vi "Decimate calc factors.vi"(9 "display width":i32, 11 "input buffer size":i32) -> (1 "decimation factor":i32, 2 "no decimation?":bool, 3 "output buffer size":i32)   [LabVIEW 2021, in "RocketPlot.lvlib"]
uses:
  RocketPlot.lvlib
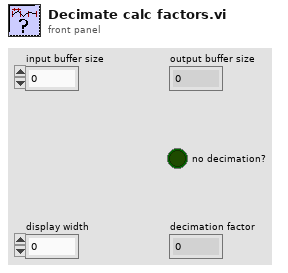
[diagram p1: front panel]
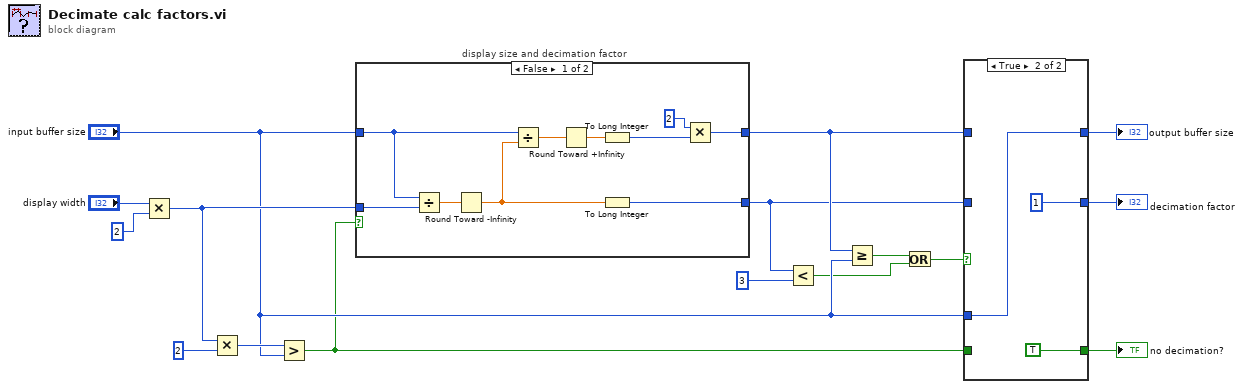
[diagram p0: block diagram]
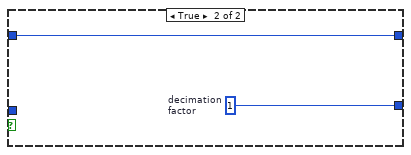
[diagram p2: hidden frame]
diagram:
  n1 = Multiply(x="display width", y=2) -> (x*y=w16:i32)
  n2 = Multiply(x=w16, y=2 ("x")) -> (x*y=w15:i32)
  n3 = Greater?(x=w15, y="input buffer size") -> (0:w1:bool)
  n4 = case "display size and decimation factor" shown="False" w1 {
    tunnel: "input buffer size" -> [w17 w28]
    tunnel: w16 -> [w26 _]
    tunnel: [w19 w28] -> w10
    tunnel: [w24 w27] -> w6
    frame False {
      n5 = Divide(x=w17, y=w26) -> (x/y=w25:dbl)
      n6 = Round Toward -Infinity(1:w25) -> (0:w23:dbl)
      n7 = Divide(x=w17, y=w23) -> (x/y=w22:dbl)
      n8 = Round Toward +Infinity(x=w22) -> (ceil(x): smallest int >= x=w21:dbl)
      n9 = To Long Integer(number=w21) -> (32bit integer=w20:i32)
      n10 = To Long Integer(number=w23) -> (32bit integer=w24:i32)
      n11 = Multiply(x=2, y=w20) -> (x*y=w19:i32)
    }
    frame True {
      w27 = 1  # decimation factor
    }
  }
  n12 = Less?(x=w6, y=3) -> (x < y?=w2:bool)
  n13 = Greater Or Equal?(x=w10, y="input buffer size") -> (x >= y?=w3:bool)
  n14 = Or(x=w3, y=w2) -> (x .or. y?=w4:bool)
  n15 = case shown="True" w4 {
    tunnel: "input buffer size" -> [_ w32]
    tunnel: w10 -> [w31 _]
    tunnel: [w31 w32] -> w9
    tunnel: w6 -> [w30 _]
    tunnel: [w30 1 ("decimation\nfactor")] -> w8
    tunnel: w1 -> [w29 _]
    tunnel: [w29 TRUE] -> w7
    frame False {
    }
    frame True {
    }
  }
  "decimation factor" <- w8
  "output buffer size" <- w9
  "no decimation?" <- w7
